vi "AddEISPotentiostatic.vi"(0 "deviceName":string, 1 "quietTimeSamplingInterval":sgl=1.0, 2 "endFreq":sgl, 3 "biasVoltage":sgl, 5 "channel":u8, 7 "repeats":u16=1, 8 "minimumCycles":u32=2, 9 "quietTime":sgl, 10 "amplitude":sgl, 11 "error in (no error)":errorcluster, 12 "startFreq":sgl, 13 "stepsPerDecade":sgl, 14 "isBiasVoltageVsOCP":bool) -> (15 "error out":errorcluster)   [LabVIEW 2018]
doc: "EXPORT void AisAddEISPotentiostatic(const char* deviceName, uint8_t channel, uint16_t repeats, float quietTime, float quietTimeSamplingInterval, float startFreq, float endFreq, float stepsPerDecade, float biasVoltage, bool isBiasVoltageVsOCP, float amplitude, unsigned int minimumCycles);"
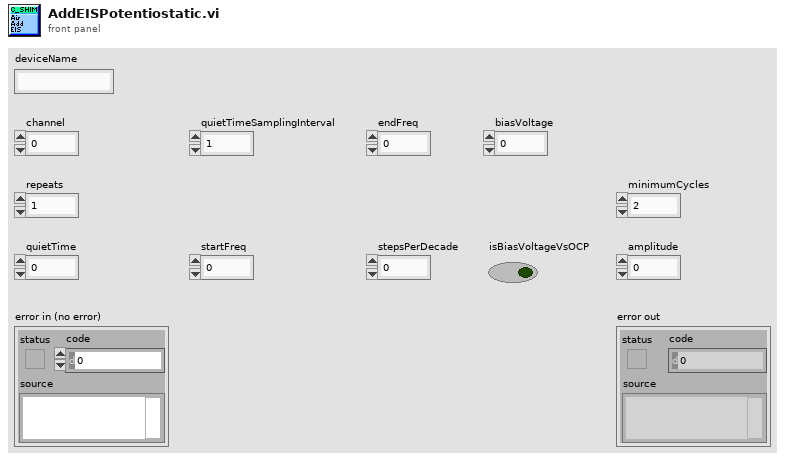
[diagram p1: front panel]
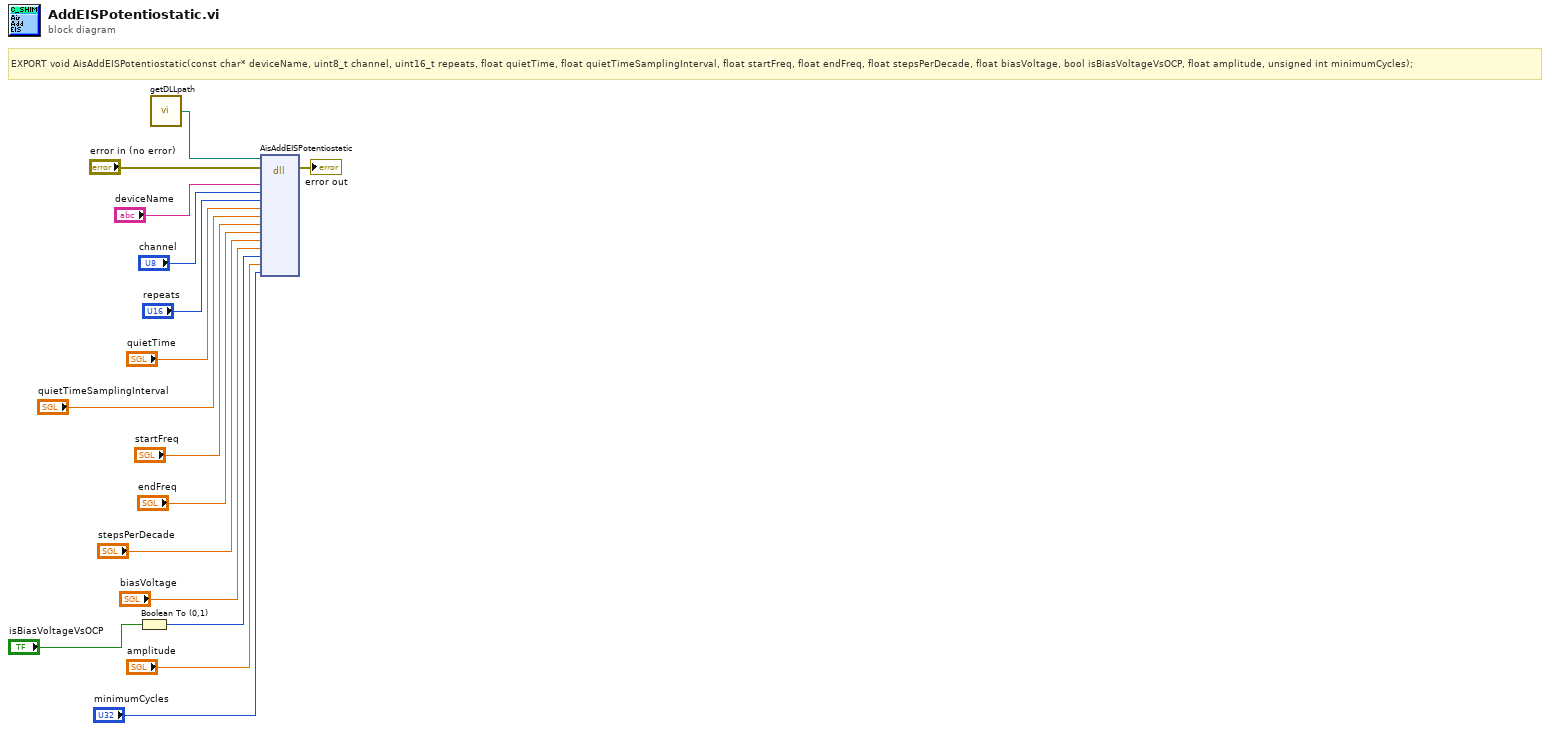
[diagram p0: block diagram]
diagram:
  # "EXPORT void AisAddEISPotentiostatic(const char* deviceName, uint8_t channel, uint16_t repeats, float quietTime, float quietTimeSamplingInterval, float startFreq, float endFreq, float stepsPerDecade, float biasVoltage, bool isBiasVoltageVsOCP, float amplitude, unsigned int minimumCycles);"
  n1 = Boolean To (0,1)(Boolean="isBiasVoltageVsOCP") -> (0, 1=w6:i16)
  n2 = call "getDLLpath.vi"() -> ("DLL_Path"=w1:path)
  n3 = dll-call lib="?" fn="AisAddEISPotentiostatic"(path in=w1, error in="error in (no error)", "deviceName"="deviceName", "channel"="channel", "repeats"="repeats", "quietTime"="quietTime", "quietTimeSamplingInterval"="quietTimeSamplingInterval", "startFreq"="startFreq", "endFreq"="endFreq", "stepsPerDecade"="stepsPerDecade", "biasVoltage"="biasVoltage", "isBiasVoltageVsOCP"=w6, "amplitude"="amplitude", "minimumCycles"="minimumCycles") -> (error out=→"error out":errorcluster)  [unwired: 14 in, 1 out]
